vi "set_voltage_channel_StreufeldDACbox.vi"(8 "error in (no error)":errorcluster, 9 "Voltage":dbl[](array[numeric]), 10 "Channel":u8[](array[numeric]), 11 "VISA Refnum in":refnum<visa-resource-name>) -> (0 "error out":errorcluster, 1 "return count":u32, 2 "Bytes at Port":u32, 3 "String":string)   [LabVIEW 2016]
uses:
  <vilib>/Instr/_visa.llb/VISA Configure Serial Port (Instr).vi
panel:
  # "SubVI to set a voltage (+-10V) on a specified channel"
  # "configured to work with the DAC-box\ncommunication via UART/COM-Port\nChannels: 1-8"
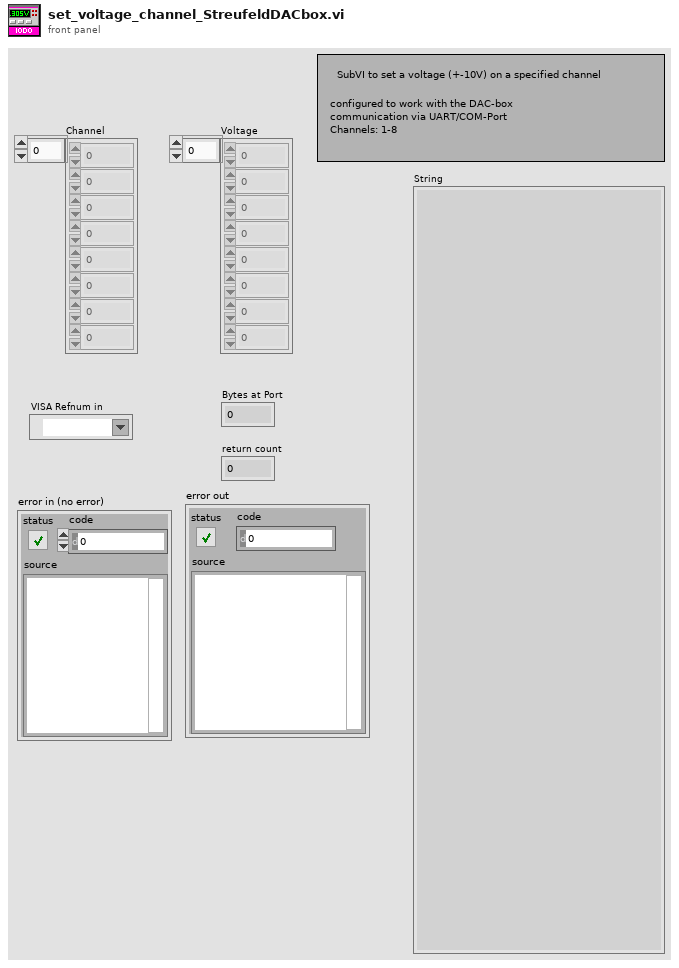
[diagram p1: front panel]
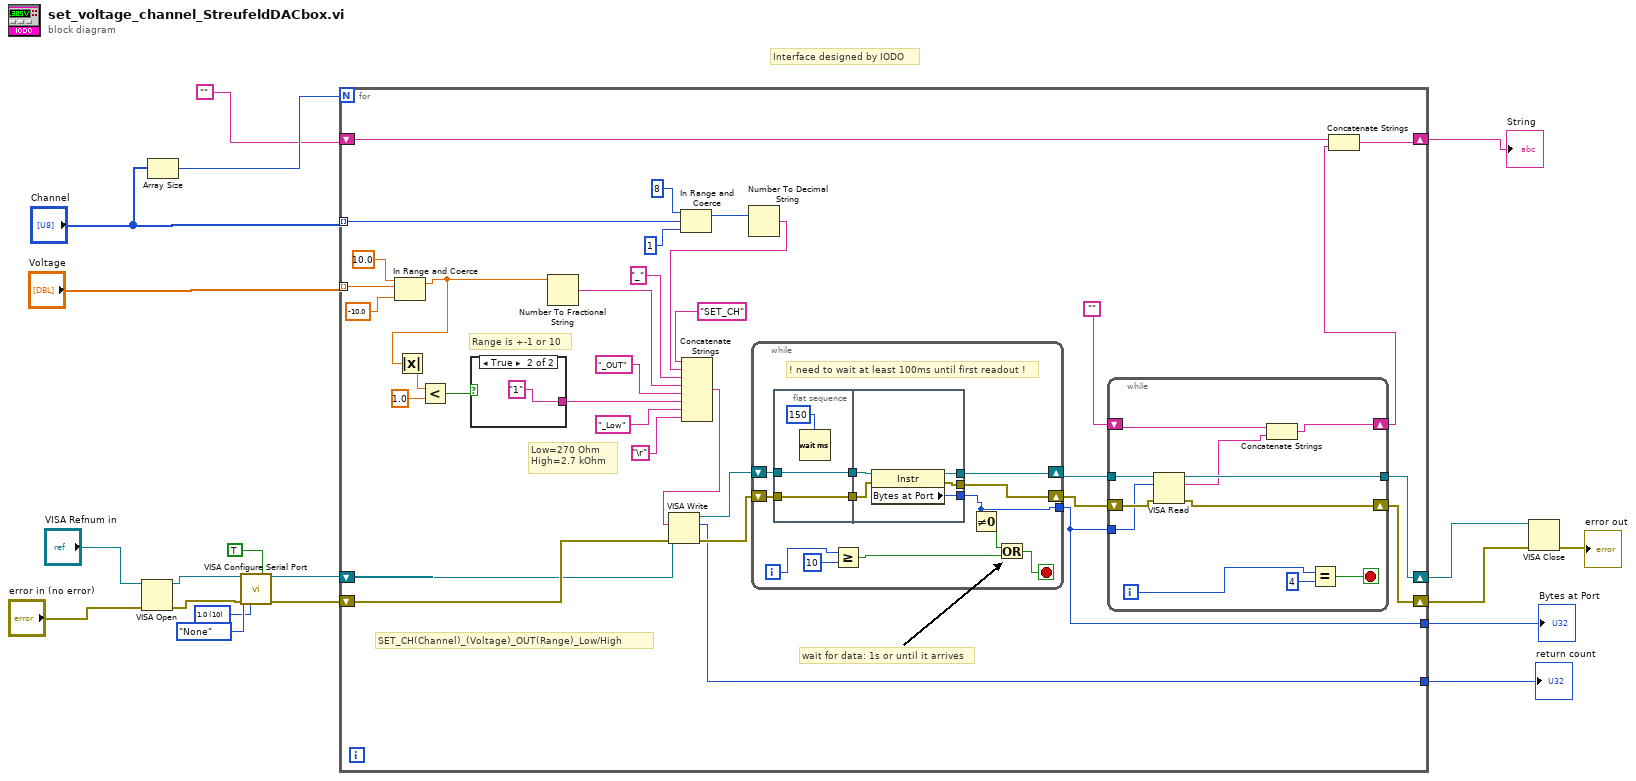
[diagram p0: block diagram]
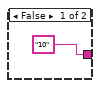
[diagram p2: hidden frame]
diagram:
  w6 = u16 10 items=["1.0"=10, "1.5"=15, "2.0"=20] ("stop bits (10: 1 bit)")
  # "Interface designed by IODO"
  n1 = VISA Open(error in (no error)="error in (no error)", VISA resource name="VISA Refnum in") -> (VISA resource name=w12:refnum<visa-resource-name>, error out=w13:errorcluster)  [unwired: 3 in]
  n2 = Array Size(array="Channel") -> (size(s)=w3:i32)
  n3 = call-poly "VISA Configure Serial Port"("VISA resource name"=w12, "Enable Termination\nChar (T)"=TRUE ("Enable Termination\nChar (T)"), "parity (0:none)"=enum16{"None", "Odd", "Even", "Mark", "Space"}."None", "error in (no error)"=w13, "stop bits (10: 1 bit)"=w6) -> ("VISA resource name out"=w10:refnum<visa-resource-name>, "error out"=w11:errorcluster)  [unwired: 9 in]
  n4 = for {
    N: w3 -> [_]
    tunnel: [w47] -> w16
    tunnel: "Voltage" -> [w42] mode=indexing
    tunnel: [w36] -> w9
    tunnel: "Channel" -> [w33] mode=indexing
    shift-right: [w49] -> w18
    shift-left: w11 -> [w38]
    shift-right: [w48] -> w17
    shift-left: w10 -> [w37]
    shift-right: [w29] -> w2
    shift-left: "" -> [w27]
    # "Low=270 Ohm\nHigh=2.7 kOhm"
    # "Range is +-1 or 10"
    # "SET_CH(Channel)_(Voltage)_OUT(Range)_Low/High"
    # "wait for data: 1s or until it arrives"
    n5 = In Range and Coerce(upper limit=10.0, x=w42, lower limit=-10.0) -> (coerced(x)=w24:dbl)  [unwired: 1 out]
    n6 = Absolute Value(x=w24) -> (abs(x)=w23:dbl)
    n7 = Less?(x=w23, y=1.0) -> (x < y?=w25:bool)
    n8 = case shown="True" w25 {
      tunnel: ["10" "1"] -> w22
      frame False {
      }
      frame True {
      }
    }
    n9 = Number To Fractional String(number=w24) -> (F-format string=w46:string)  [unwired: 3 in]
    n10 = In Range and Coerce(upper limit=u8 8, x=w33, lower limit=u8 1) -> (coerced(x)=w32:u8)  [unwired: 1 out]
    n11 = Number To Decimal String(number=w32) -> (decimal integer string=w53:string)  [unwired: 1 in]
    n12 = Concatenate Strings("SET_CH" ("write buffer"), w53, "_" ("string"), w46, "_OUT" ("string"), w22, "_Low" ("string"), "\r") -> (w41:string)
    n13 = VISA Write(VISA resource name=w37, write buffer=w41, error in (no error)=w38) -> (VISA resource name out=w39:refnum<visa-resource-name>, return count=w36:u32, error out=w40:errorcluster)
    n14 = while {
      shift-right: [w69] -> w34
      shift-left: w39 -> [w72]
      shift-right: [w68] -> w35
      shift-left: w40 -> [w70]
      tunnel: [w67] -> w47
      i -> [w78]
      stop <- w74 stop-if-true
      # "! need to wait at least 100ms until first readout !"
      n15 = flat-sequence {
        tunnel: [w80] -> w73
        tunnel: w72 -> [w80]
        tunnel: [w79] -> w71
        tunnel: w70 -> [w79]
        tunnel: w73 -> [w86]
        tunnel: w71 -> [w85]
        tunnel: [w84] -> w69
        tunnel: [w83] -> w68
        tunnel: [w82] -> w67
        frame #0 {
          n16 = Wait (ms)(milliseconds to wait=u32 150) -> ()  [unwired: 1 out]
        }
        frame #1 {
          n17 = property class="Instr"(reference=w86, error in=w85) -> (reference out=w84:refnum<visa-resource-name>, error out=w83:errorcluster, "Bytes at Port"=w82:u32)
        }
      }
      n18 = Greater Or Equal?(x=w78, y=10) -> (x >= y?=w76:bool)
      n19 = Not Equal To 0?(x=w67) -> (x != 0?=w75:bool)
      n20 = Or(x=w75, y=w76) -> (x .or. y?=w74:bool)
    }
    n21 = while {
      tunnel: w34 -> [w66]
      tunnel: w47 -> [w64]
      shift-right: [w62] -> w28
      shift-left: "" -> [w63]
      tunnel: [w61] -> w48
      shift-right: [w60] -> w49
      shift-left: w35 -> [w65]
      i -> [w58]
      stop <- w57 stop-if-true
      n22 = VISA Read(VISA resource name=w66, byte count=w64, error in (no error)=w65) -> (VISA resource name out=w61:refnum<visa-resource-name>, read buffer=w59:string, error out=w60:errorcluster)  [unwired: 1 out]
      n23 = Concatenate Strings(w63, w59) -> (w62:string)
      n24 = Equal?(x=w58, y=4) -> (x = y?=w57:bool)
    }
    n25 = Concatenate Strings(w27, w28) -> (w29:string)
  }
  "String" <- w2
  "Bytes at Port" <- w16
  "return count" <- w9
  n26 = VISA Close(VISA resource name=w17, error in (no error)=w18) -> (error out=→"error out":errorcluster)
